vi "SR2000Read.vi"(8 "error in (no error)":errorcluster, 11 "Data In":T1) -> (0 "error out":errorcluster, 2 "BarCodeRead":string, 3 "Data Out":T1)   [LabVIEW 2014]
uses:
  controls/Data1.ctl
  controls/Payjson.ctl
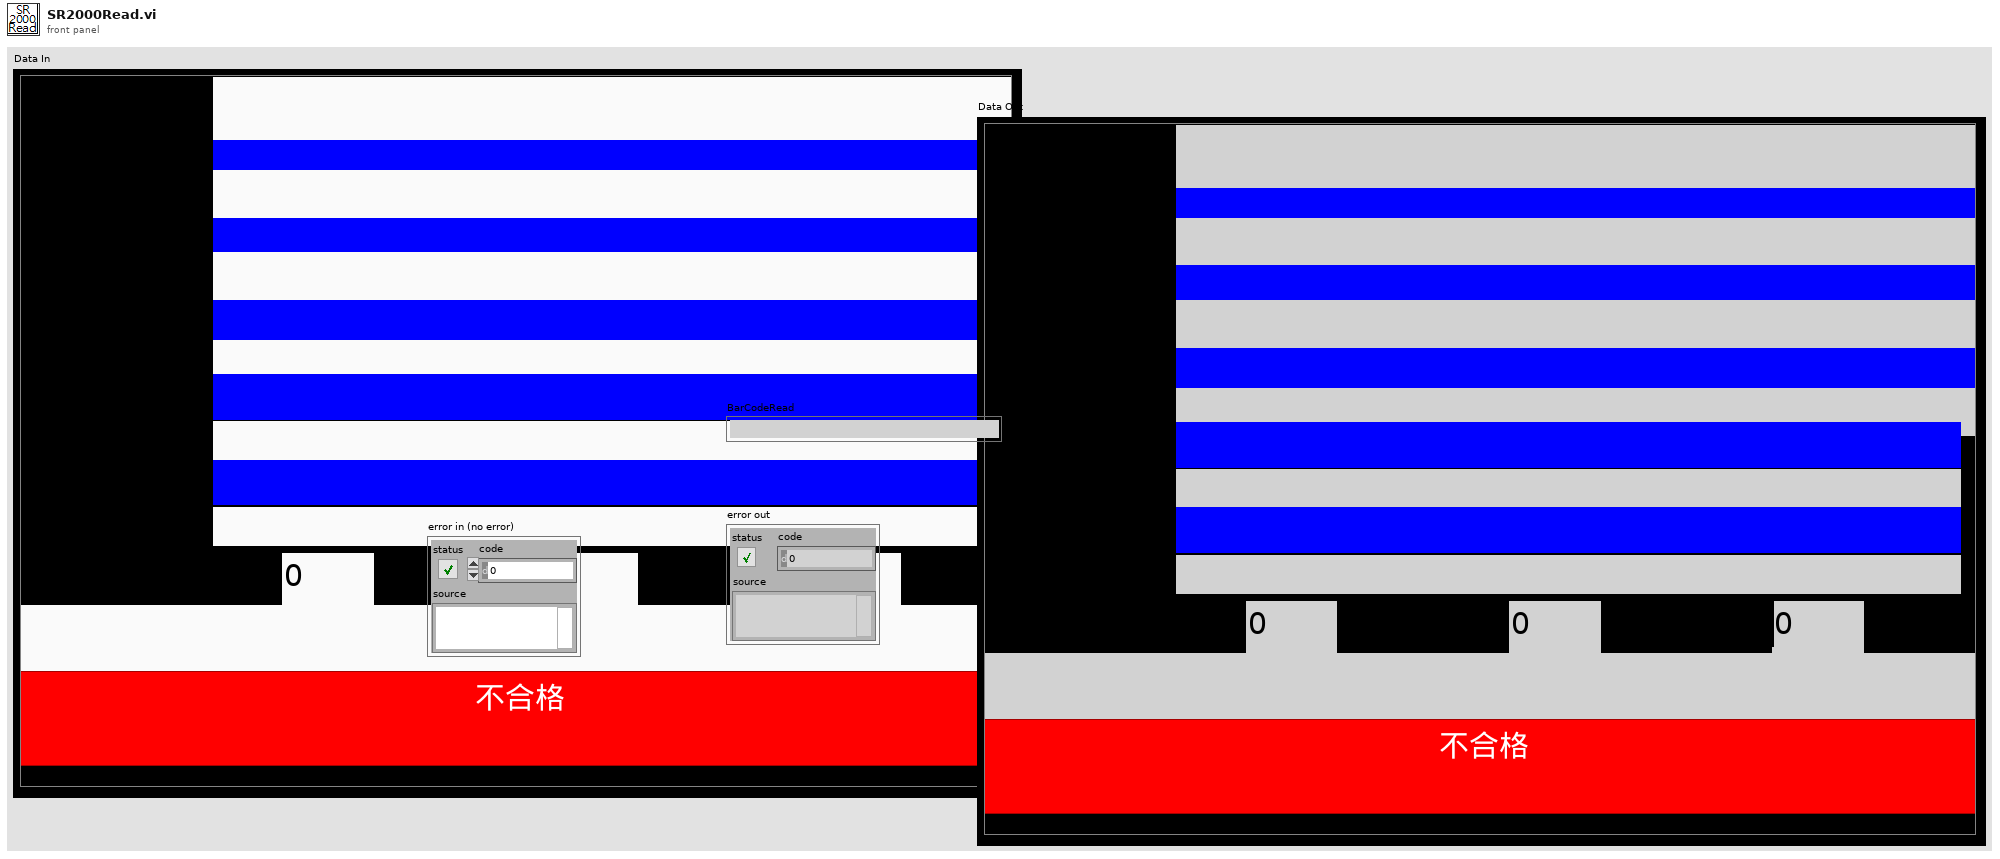
[diagram p1: front panel]
types:
  T1 = typedef "Data1.ctl" = cluster{"Date":string, "BarCode1":string, "BarCode2":string, "BarCode3":string, "Message":string, "OK Count":u16, "NG Count":u16, "Total Count":u16, "ModelData":string[][], "OK&NG":bool, "COM1":refnum<visa-resource-name>, "COM2":refnum<visa-resource-name>, "IO":i32, "Time":u32, "TCP":refnum<k5>, "TCP 2":refnum<k5>, "COM1 2":refnum<visa-resource-name>, "CheckNum":string, "BarCode1_1":string, "BarCode2_1":string, "BarCode3_1":string, "日期":string, "機種":string, "機號":string, "商品條碼1":string, "OK_1":string, "OK":string, "NG":string, "NG_1":string, "Total":string, "Total_1":string, "ClaerTime":u32, "Pjson":T2, "LotNo":string[], "CheckParsArray":string[], "BarCode4":string, "BarCode4_1":string, "商品條碼2":string, "BarCode5":string, "BarCode5_1":string, "商品條碼3":string, "ReScanNG":i32, "NGTimeCT":u32}
  T2 = typedef "Payjson.ctl" = cluster{"DEPT":string, "LINE":string, "STANO":string, "WORKNO":string, "PRODSN":string, "COMPNTID":string, "COMPNTLOT":string, "COMPNTSN":string, "USEDQTY":i16, "OPDATE":string, "OPUSER":string, "RECVDATE":string, "MMODU":string}[]
  T3 = typedef "Data.ctl" = cluster{"Date":string, "BarCode1":string, "BarCode2":string, "BarCode3":string, "Message":string, "OK Count":u16, "NG Count":u16, "Total Count":u16, "ModelData":string[][], "OK&NG":bool, "COM1":refnum<visa-resource-name>, "COM2":refnum<visa-resource-name>, "IO":i32, "Time":u32, "TCP":refnum<k5>, "TCP 2":refnum<k5>, "COM3":refnum<visa-resource-name>, "CheckPars":string}
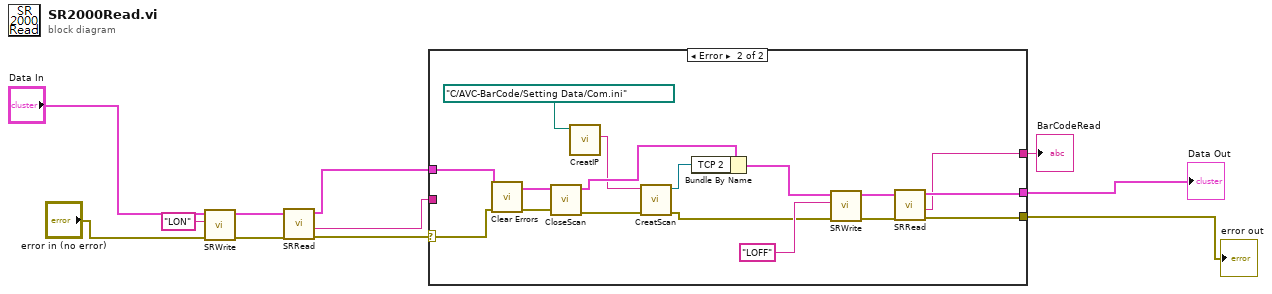
[diagram p0: block diagram]
diagram:
  n1 = call "SRWrite.vi"("error in (no error)"="error in (no error)", "Command"="LON", "Data In"="Data In") -> ("error out"=w10:errorcluster, "Data Out"=w11:T3)  [unwired: 7 in]
  n2 = call "SRRead.vi"("error in (no error)"=w10, "Data In"=w11) -> ("error out"=w8:errorcluster, "BarCodeRead"=w6:string, "Data Out"=w7:T3)  [unwired: 7 in]
  n3 = case shown="Error" w8 {
    selector: w8 -> [w12 w30]
    tunnel: w7 -> [w13 w27]
    tunnel: [w14 w17] -> w5
    tunnel: w6 -> [w14 _]
    tunnel: [w13 w20] -> w3
    tunnel: [w12 w18] -> w1
    frame No Error {
    }
    frame Error {
      n4 = call <vilib>:"Clear Errors.vi"("error in (no error)"=w30) -> ("error out"=w28:errorcluster)  [unwired: 5 in, 1 out]
      n5 = call "CloseScan.vi"("error in (no error)"=w28, "Data In"=w27) -> ("error out"=w25:errorcluster, "Data Out"=w26:T1)  [unwired: 8 in]
      n6 = call "CreatIP.vi"("file Path"=path "C:/AVC-BarCode/Setting Data/Com.ini") -> ("Scan IP"=w15:string)  [unwired: 7 in, 3 out]
      n7 = call "CreatScan.vi"("error in (no error)"=w25, "address"=w15) -> ("error out"=w22:errorcluster, "TCP Out"=w29:refnum<k5>)  [unwired: 7 in, 1 out]
      n8 = Bundle By Name(cluster=w26, "TCP 2"=w29) -> (w23:T1)
      n9 = call "SRWrite.vi"("error in (no error)"=w22, "Command"="LOFF", "Data In"=w23) -> ("error out"=w19:errorcluster, "Data Out"=w21:T3)  [unwired: 7 in]
      n10 = call "SRRead.vi"("error in (no error)"=w19, "Data In"=w21) -> ("error out"=w18:errorcluster, "BarCodeRead"=w17:string, "Data Out"=w20:T3)  [unwired: 7 in]
    }
  }
  "Data Out" <- w3
  "BarCodeRead" <- w5
  "error out" <- w1
